vi "group Sync Read Remove Param.vi"(10 "id":u8, 11 "group_num":i32) -> ()   [LabVIEW 2016, in "dxl_x86_c.lvlib"]
doc: "WINDECLSPEC void groupSyncReadRemoveParam (int group_num, uint8_t id);"
uses:
  dxl_x86_c.lvlib
  dxl_x86_c.dll
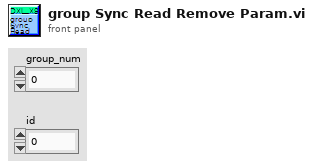
[diagram p1: front panel]
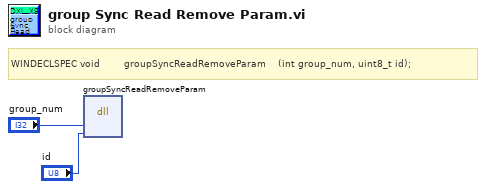
[diagram p0: block diagram]
diagram:
  # "WINDECLSPEC void        groupSyncReadRemoveParam    (int group_num, uint8_t id);"
  n1 = dll-call lib="C:/Users/Platform/Desktop/DynamixelSDK/labview/dxl_x86_c.lvlib/dxl_x86_c.*" fn="groupSyncReadRemoveParam"("group_num"="group_num", "id"="id") -> ()  [unwired: 6 in, 2 out]
